vi "写入数据库.vi"(7 "table输入":string, 8 "error in (no error)":errorcluster, 9 "数据标记表":string(combo)="N", 10 "测量模式":T2(ring)=enum."水样测试", 11 "data in":T1) -> (0 "error out":errorcluster)   [LabVIEW 2016, in "HACH多参.lvlib"]
uses:
  <vilib>/Utility/sysdir.llb/System Directory Type.ctl
  <vilib>/addons/database/Connection.llb/DB Tools Open Connec (String).vi
  <vilib>/addons/database/NI_Database_API.lvlib
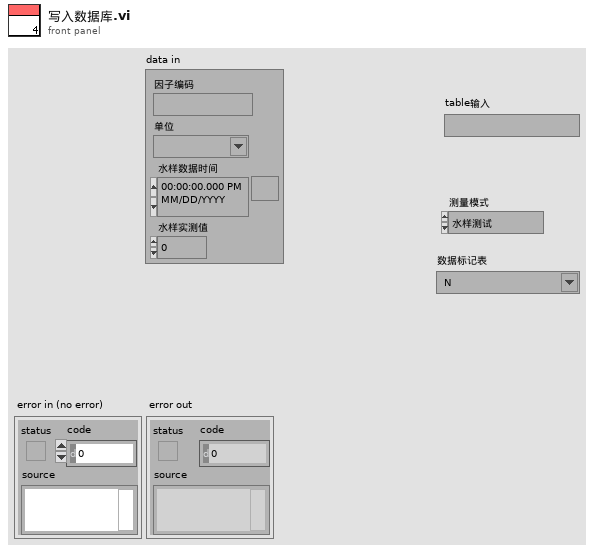
[diagram p1: front panel]
types:
  T1 = cluster{"因子编码":string, "单位":string, "水样数据时间":timestamp, "水样实测值":sgl}
  T2 = enum16{"待机", "水样测试", "标样核查", "零点核查", "跨度核查", "空白测试", "平行样测试", "加标回收", "空白校准", "标样校准", "初始化（清洗）"}
  T3 = cluster{"时间标识":timestamp, "测量模式":string, "数据类型":string, "监测值":sgl, "单位":string, "数据标识":string, "因子编码":string, "标样参考值":dbl}
  T4 = typedef "System Directory Type.ctl" = i32
  T5 = typedef "NI_Database_API.lvlib/Conn ObjectReference.ctl" = refnum<k1>
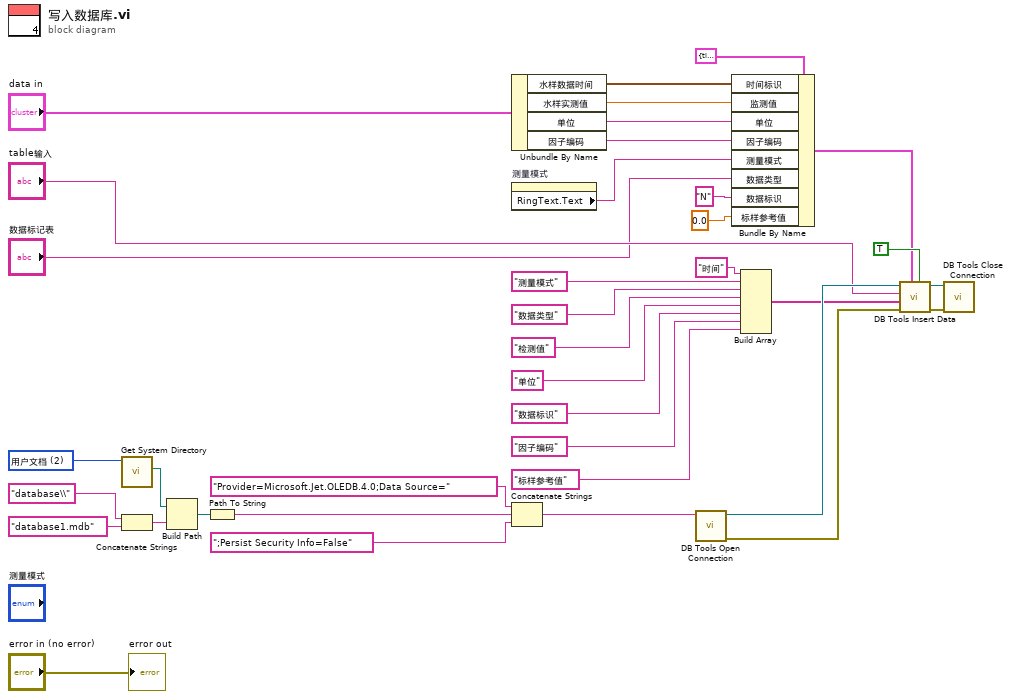
[diagram p0: block diagram]
diagram:
  w24 = T4 2 items=["用户目录"=0, "用户桌面"=1, "用户文档"=2, "用户应用程序数据"=3, "用户设置"=4, "用户临时目录"=5, "公共文档"=6, "公共应用程序数据"=7, "公共设置"=8, "公共缓存"=13, "系统核心库"=9, "系统安装库"=10, "应用程序文件"=11, "启动盘根目录"=12] ("system directory type")
  n1 = call <vilib>:"Get System Directory.vi"("system directory type"=w24) -> ("system directory"=w22:path)  [unwired: 10 in]
  n2 = Concatenate Strings("database\\" ("condition"), "database1.mdb" ("字符串")) -> (w16:string)
  n3 = Build Path(base path=w22, name or relative path=w16) -> (appended path=w21:path)
  n4 = Path To String(path=w21) -> (string=w20:string)
  n5 = Unbundle By Name("data in") -> ("水样数据时间"=w34:timestamp, "水样实测值"=w33:sgl, "单位"=w32:string, "因子编码"=w7:string)
  n6 = property on="测量模式" class="Enum (严格)"() -> ("RingText.Text"=w31:string)  [unwired: 2 in, 2 out]
  n7 = Concatenate Strings("Provider=Microsoft.Jet.OLEDB.4.0;Data Source=" ("condition"), w20, ";Persist Security Info=False" ("condition")) -> (w18:string)
  n8 = call-poly <vilib>:"DB Tools Open Connection.vi"("connection information"=w18) -> ("error out"=w14:errorcluster, "connection reference"=w15:T5)  [unwired: 7 in]
  n9 = Bundle By Name(cluster=T3 {"时间标识"=timestamp(0 s since 1904-01-01), "测量模式"="", "数据类型"="", "监测值"=0.0, "单位"="", "数据标识"="", "因子编码"="", "标样参考值"=0.0} ("data输出"), "时间标识"=w34, "监测值"=w33, "单位"=w32, "因子编码"=w7, "测量模式"=w31, "数据类型"="数据标记表", "数据标识"="N", "标样参考值"=0.0) -> (w11:T3)
  n10 = Build Array("时间", "测量模式", "数据类型", "检测值", "单位", "数据标识", "因子编码", "标样参考值") -> (w12:string[])
  n11 = call <vilib>:"DB Tools Insert Data.vi"("create table? (F)"=TRUE, "data"=w11, "error in (no error)"=w14, "columns"=w12, "table"="table输入", "connection reference"=w15) -> ("error out"=w26:errorcluster, "connection reference out"=w27:T5)  [unwired: 4 in]
  n12 = call <vilib>:"DB Tools Close Connection.vi"("error in (no error)"=w26, "connection reference"=w27) -> ()  [unwired: 5 in, 1 out]
  "error out" <- "error in (no error)"
